vi "Calculate position from parameters.vi"(6 "Current step":dbl, 8 "error in (no error)":errorcluster, 9 "°/step":dbl, 10 "Step style motor":T1=1 items=["", "Single", "Double", "Interleave", "Microstep"], 11 "Motor direction":T2 items=["", "Forward", "Backward"]) -> (0 "error out":errorcluster, 3 "Position adjustment":dbl)   [LabVIEW 2020, in "Control de MaP.lvlib"]
uses:
  Control de MaP.lvlib
  Controls/Motor direction.ctl
  Controls/Step style.ctl
  Arduino-Adafruit stepper/Arduino-Adafruit stepper.lvlib
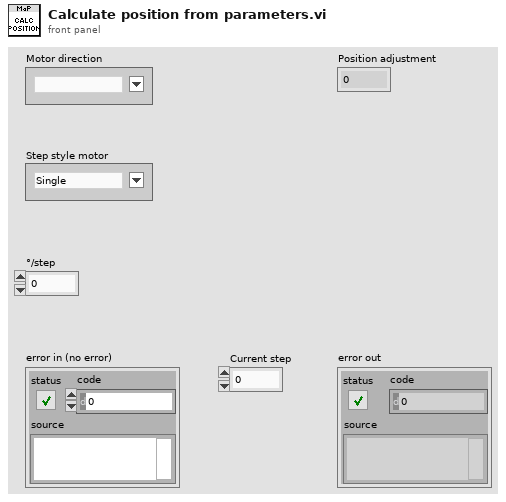
[diagram p1: front panel]
types:
  T1 = typedef "Arduino-Adafruit stepper.lvlib/Step style.ctl" = u8
  T2 = typedef "Arduino-Adafruit stepper.lvlib/Motor direction.ctl" = u8
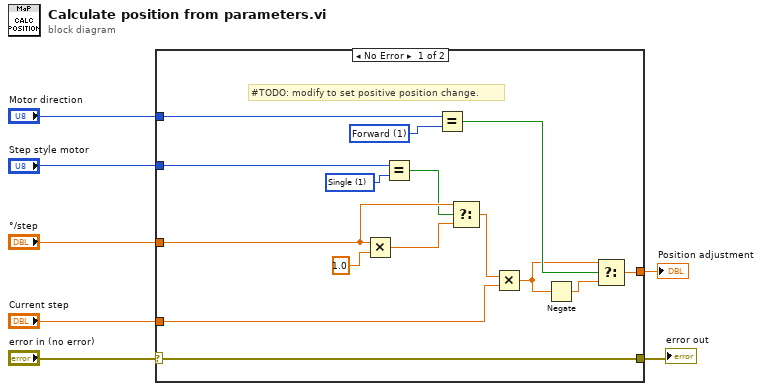
[diagram p0: block diagram]
diagram:
  n1 = case shown="No Error" "error in (no error)" {
    selector: "error in (no error)" -> [w12 w23]
    tunnel: "°/step" -> [w20 _]
    tunnel: [w19 w24] -> w6
    tunnel: "Motor direction" -> [w17 _]
    tunnel: "Step style motor" -> [w14 _]
    tunnel: "Current step" -> [w13 w24]
    tunnel: [w12 w23] -> w2
    frame No Error {
      w10 = T1 1 items=["", "Single", "Double", "Interleave", "Microstep"] ("Step style motor")
      w11 = T2 1 items=["", "Forward", "Backward"] ("Motor direction")
      # "#TODO: modify to set positive position change."
      n2 = Multiply(x=w20, y=1.0) -> (x*y=w22:dbl)
      n3 = Equal?(x=w14, y=w10) -> (x = y?=w15:bool)
      n4 = Equal?(x=w17, y=w11) -> (x = y?=w18:bool)
      n5 = Select(t=w20, s=w15, f=w22) -> (s? t:f=w16:dbl)
      n6 = Multiply(x=w16, y=w13) -> (x*y=w8:dbl)
      n7 = Negate(x=w8) -> (-x=w9:dbl)
      n8 = Select(t=w8, s=w18, f=w9) -> (s? t:f=w19:dbl)
    }
    frame Error {
    }
  }
  "Position adjustment" <- w6
  "error out" <- w2
